vi "Bootloader - Send Packet.vi"(0 "VISA resource name":refnum<visa-resource-name>, 2 "Data Fixed Length":i32, 5 "Address":u32, 7 "Data Length":u32, 9 "Data":u8[](array[numeric]) format="%.0x", 11 "error in (no error)":errorcluster, 13 "Op Code":u16(ring) items=["Write Page"=0, "Write EEPROM"=2, "Read EEPROM"=3, "Get Page Size"=102, "Leave Bootloader"=119]) -> (4 "VISA resource name":refnum<visa-resource-name>, 6 "Address":u32, 8 "Data Length":u32, 10 "Data":u8[](array[numeric]) format="%.0x", 15 "error out":errorcluster)   [LabVIEW 2010]
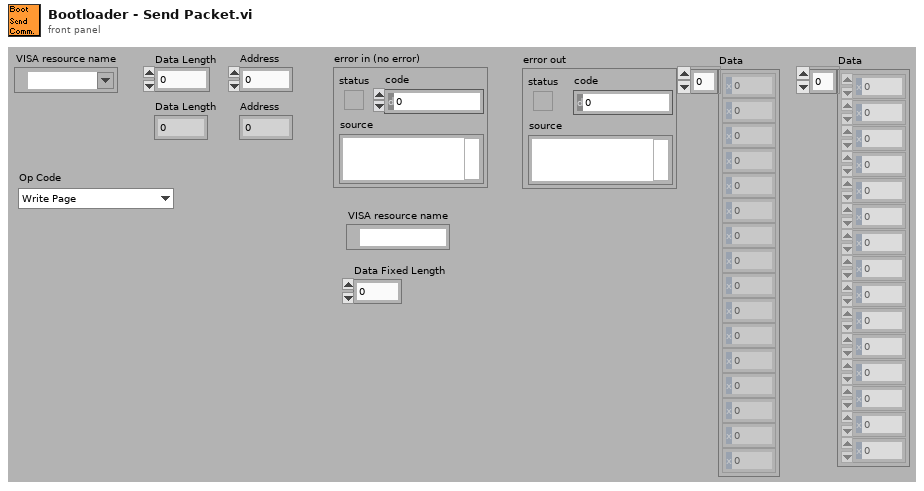
[diagram p1: front panel]
types:
  T1 = enum16{"big-endian, network order", "native, host order", "little-endian"}
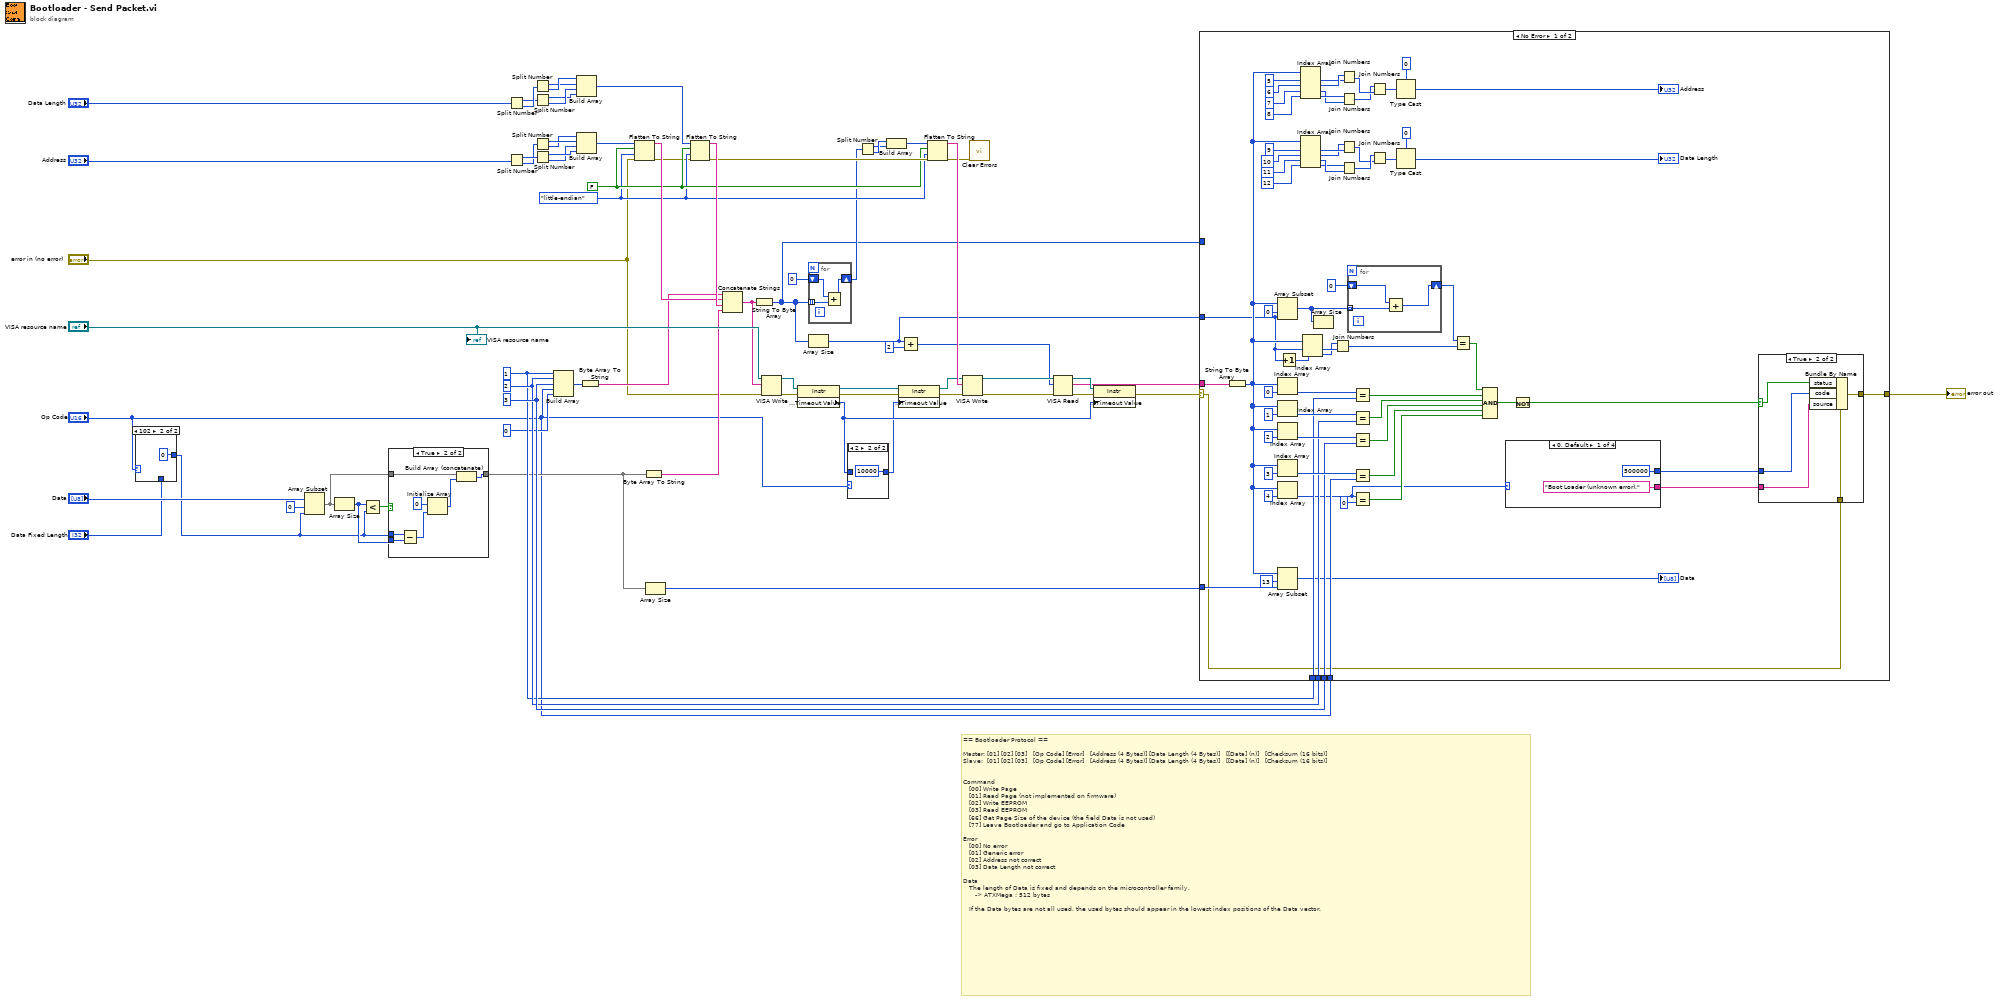
[diagram p0: block diagram]
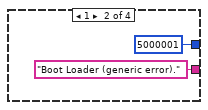
[diagram p5: hidden frame]
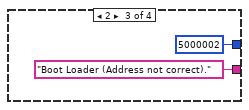
[diagram p6: hidden frame]
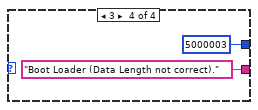
[diagram p7: hidden frame]
diagram:
  w54 = T1."little-endian" ("byte order (0:big-endian, network order)")
  w55 = FALSE ("prepend array or string size? (T)")
  w62 = u8 3 ("element")
  w61 = u8 2 ("element")
  w60 = u8 1 ("element")
  # "== Bootloader Protocol ==\n\nMaster: [01] [02] [03]   [Op Code] [Error]   [Address (4 Bytes)] [Data Length (4 Bytes)]   [[Data] (n)]   [Checksum (16 bits)]\nSlave:  [01] [02] [03]   [Op Code] [Error]   [Address (4 Bytes)] [Data Length (4 Bytes)]   [[Data] (n)]   [Checksum (16 bits)]\n\n\nCommand\n   [00] Write Page\n   [01] Read Page (not implemented on firmware)\n   [02] Write EEPROM\n   [03] Read EEPROM\n   [66] Get Page Size of the device (the field Data is not used)\n   [77] Leave Bootloader and go to Application Code\n\nError\n   [00] No error\n   [01] Generic error\n   [02] Address not correct\n   [03] Data Length not correct\n\nData\n   The length of Data is fixed and depends on the microcontroller family.\n      -> ATXMega : 512 bytes\n\n   If the Data bytes are not all used, the used bytes should appear in the lowest index positions of the Data vector."
  n1 = case shown="102" "Op Code" {
    tunnel: [w69 0 ("Timeout")] -> w3
    tunnel: "Data Fixed Length" -> [w69 _]
    frame 0, Default {
    }
    frame 102 {
    }
  }
  n2 = Array Subset(array="Data", index=0, length=w3) -> (w21:u8[])
  n3 = Array Size(array=w21) -> (size(s)=w20:i32)
  n4 = Less?(x=w20, y=w3) -> (x < y?=w22:bool)
  n5 = case shown="True" w22 {
    tunnel: w21 -> [w71 w74]
    tunnel: w3 -> [_ w78]
    tunnel: w20 -> [_ w77]
    tunnel: [w71 w73] -> w18
    frame False {
    }
    frame True {
      n6 = Subtract(x=w78, y=w77) -> (x-y=w76:i32)
      n7 = Initialize Array(u8 0 ("element"), w76) -> (w75:u8[])
      n8 = Build Array (concatenate)(w74, w75) -> (w73:u8[])
    }
  }
  n9 = Split Number(x="Data Length") -> (hi(x)=w41:u16, lo(x)=w42:u16)
  n10 = Split Number(x="Address") -> (hi(x)=w36:u16, lo(x)=w35:u16)
  n11 = Split Number(x=w42) -> (hi(x)=w43:u8, lo(x)=w44:u8)
  n12 = Split Number(x=w41) -> (hi(x)=w39:u8, lo(x)=w40:u8)
  n13 = Split Number(x=w35) -> (hi(x)=w34:u8, lo(x)=w33:u8)
  n14 = Split Number(x=w36) -> (hi(x)=w38:u8, lo(x)=w37:u8)
  n15 = Build Array(w60, w61, w62, "Op Code", u8 0 ("element")) -> (w48:u16[])
  n16 = Build Array(w44, w43, w40, w39) -> (w46:u8[])
  n17 = Build Array(w33, w34, w37, w38) -> (w32:u8[])
  n18 = Byte Array To String(unsigned byte array=w48) -> (string=w63:string)
  n19 = Flatten To String(anything=w32, prepend array or string size? (T)=w55, byte order (0:big-endian, network order)=w54, error in (no error)="error in (no error)") -> (data string=w64:string, error out=w45:errorcluster)  [unwired: 1 out]
  n20 = Byte Array To String(unsigned byte array=w18) -> (string=w30:string)
  n21 = Array Size(array=w18) -> (size(s)=w28:i32)
  n22 = Flatten To String(anything=w46, prepend array or string size? (T)=w55, byte order (0:big-endian, network order)=w54, error in (no error)=w45) -> (data string=w65:string, error out=w56:errorcluster)  [unwired: 1 out]
  n23 = Concatenate Strings(w63, w64, w65, w30) -> (w66:string)
  n24 = String To Byte Array(string=w66) -> (unsigned byte array=w26:u8[])
  n25 = VISA Write(VISA resource name="VISA resource name", write buffer=w66, error in (no error)="error in (no error)") -> (VISA resource name out=w15:refnum<visa-resource-name>, error out=w16:errorcluster)  [unwired: 1 out]
  n26 = property class="Instr"(reference=w15, error in=w16) -> (reference out=w11:refnum<visa-resource-name>, error out=w12:errorcluster, "General Settings:Timeout Value"=w8:u32)
  n27 = Array Size(array=w26) -> (size(s)=w25:i32)
  n28 = for {
    tunnel: w26 -> [w81] mode=indexing
    shift-right: [w79] -> w53
    shift-left: u16 0 ("page address") -> [w80]
    n29 = Add(x=w80, y=w81) -> (x+y=w79:u16)
  }
  n30 = case shown="2" "Op Code" {
    tunnel: w8 -> [w82 _]
    tunnel: [w82 u32 10000 ("Timeout")] -> w7
    frame 0, Default {
    }
    frame 2 {
    }
  }
  n31 = Split Number(x=w53) -> (hi(x)=w50:u8, lo(x)=w51:u8)
  n32 = Build Array(w51, w50) -> (w52:u8[])
  n33 = property class="Instr"(reference=w11, error in=w12, "General Settings:Timeout Value"=w7) -> (reference out=w13:refnum<visa-resource-name>, error out=w14:errorcluster)
  n34 = Add(x=w25, y=2) -> (x+y=w27:i32)
  n35 = Flatten To String(anything=w52, prepend array or string size? (T)=w55, byte order (0:big-endian, network order)=w54, error in (no error)=w56) -> (data string=w58:string, error out=w57:errorcluster)  [unwired: 1 out]
  n36 = VISA Write(VISA resource name=w13, write buffer=w58, error in (no error)=w14) -> (VISA resource name out=w59:refnum<visa-resource-name>, error out=w6:errorcluster)  [unwired: 1 out]
  n37 = call <vilib>:"Clear Errors.vi"("error in (no error)"=w57) -> ()  [unwired: 6 in, 1 out]
  n38 = VISA Read(VISA resource name=w59, byte count=w27, error in (no error)=w6) -> (VISA resource name out=w10:refnum<visa-resource-name>, read buffer=w1:string, error out=w9:errorcluster)  [unwired: 1 out]
  n39 = property class="Instr"(reference=w10, error in=w9, "General Settings:Timeout Value"=w8) -> (error out=w5:errorcluster)  [unwired: 1 out]
  n40 = case shown="No Error" w5 {
    selector: w5 -> [w89 w168]
    tunnel: w1 -> [w150 _]
    tunnel: w60 -> [w140 _]
    tunnel: w61 -> [w139 _]
    tunnel: w62 -> [w138 _]
    tunnel: "Op Code" -> [w137 _]
    tunnel: [w87 w168] -> w67
    tunnel: w28 -> [w97 _]
    tunnel: w25 -> [w93 _]
    tunnel: w26 -> [_ _]
    frame No Error {
      n41 = String To Byte Array(string=w150) -> (unsigned byte array=w95:u8[])
      n42 = Array Subset(array=w95, index=0, length=w93) -> (w94:u8[])
      n43 = Index Array(array=w95, index=0) -> (element=w144:u8)
      n44 = Index Array(array=w95, index=1) -> (element=w143:u8)
      n45 = Index Array(array=w95, index=2) -> (element=w142:u8)
      n46 = Index Array(array=w95, index=3) -> (element=w141:u8)
      n47 = Index Array(array=w95, index=4) -> (element=w86:u8)
      n48 = Array Subset(array=w95, index=13, length=w97) -> (→"Data":u8[])
      n49 = Increment(x=w93) -> (x+1=w92:i32)
      n50 = Index Array(array=w95, index #1=5 ("index"), index #2=6 ("index"), index #3=7 ("index"), index #4=8 ("index")) -> (element #1=w117:u8, element #2=w121:u8, element #3=w118:u8, element #4=w119:u8)
      n51 = Index Array(array=w95, index #1=9 ("index"), index #2=10 ("index"), index #3=11 ("index"), index #4=12 ("index")) -> (element #1=w108:u8, element #2=w104:u8, element #3=w107:u8, element #4=w106:u8)
      n52 = Index Array(array=w95, index #1=w93, index #2=w92) -> (element #1=w91:u8, element #2=w90:u8)
      n53 = Array Size(array=w94) -> ()  [unwired: 1 out]
      n54 = Join Numbers(hi=w90, lo=w91) -> ((hi.lo)=w128:u16)
      n55 = Join Numbers(hi=w121, lo=w117) -> ((hi.lo)=w122:u16)
      n56 = Join Numbers(hi=w119, lo=w118) -> ((hi.lo)=w120:u16)
      n57 = Join Numbers(hi=w104, lo=w108) -> ((hi.lo)=w103:u16)
      n58 = Join Numbers(hi=w106, lo=w107) -> ((hi.lo)=w105:u16)
      n59 = for {
        tunnel: w94 -> [w167] mode=indexing
        shift-right: [w165] -> w127
        shift-left: u16 0 ("page address") -> [w166]
        n60 = Add(x=w166, y=w167) -> (x+y=w165:u16)
      }
      n61 = Equal?(x=w144, y=w140) -> (x = y?=w136:bool)
      n62 = Equal?(x=w143, y=w139) -> (x = y?=w135:bool)
      n63 = Equal?(x=w142, y=w138) -> (x = y?=w134:bool)
      n64 = Equal?(x=w141, y=w137) -> (x = y?=w133:bool)
      n65 = Equal?(x=w86, y=u8 0) -> (x = y?=w131:bool)
      n66 = Join Numbers(hi=w120, lo=w122) -> ((hi.lo)=w123:u32)
      n67 = Join Numbers(hi=w105, lo=w103) -> ((hi.lo)=w102:u32)
      n68 = Type Cast(type=u32 0 ("byte count"), x=w123) -> (*(type *) &x=→"Address":u32)
      n69 = Type Cast(type=u32 0 ("byte count"), x=w102) -> (*(type *) &x=→"Data Length":u32)
      n70 = Equal?(x=w127, y=w128) -> (x = y?=w126:bool)
      n71 = Compound Arithmetic op=AND(w126, w136, w135, w134, w133, w131) -> (w125:bool)
      n72 = case shown="0, Default" w86 {
        tunnel: ["Boot Loader (unknown error)." ("source") "Boot Loader (generic error)." ("source") "Boot Loader (Address not correct)." ("source") "Boot Loader (Data Length not correct)." ("source")] -> w85
        tunnel: [500000 ("code") 5000001 ("code") 5000002 ("code") 5000003 ("code")] -> w84
        frame 0, Default {
        }
        frame 1 {
        }
        frame 2 {
        }
        frame 3 {
        }
      }
      n73 = Not(x=w125) -> (.not. x?=w88:bool)
      n74 = case shown="True" w88 {
        selector: w88 -> [_ w162]
        tunnel: w89 -> [w159 w164]
        tunnel: [w159 w163] -> w87
        tunnel: w85 -> [_ w161]
        tunnel: w84 -> [_ w160]
        frame False {
        }
        frame True {
          n75 = Bundle By Name(cluster=w164, "status"=w162, "code"=w160, "source"=w161) -> (w163:errorcluster)
        }
      }
    }
    frame Error {
    }
  }
  "error out" <- w67
  "VISA resource name" <- "VISA resource name"
